vi "RT Loop - Acquire camera_data_1.vi"(8 "Boolean":bool, 11 "Message Queue":refnum<queue>) -> ()   [LabVIEW 2017]
uses:
  UI Error Handlers/support/Message Queue/Message Cluster.ctl
  <vilib>/userdefined/High Color/IMAQdx.ctl
  <vilib>/vision/Avi.llb/IMAQ AVI2 Codec Path.ctl
  <vilib>/vision/Avi.llb/IMAQ AVI2 Refnum.ctl
  Globals/Global - All RT Loop Stop.vi
  Globals/Global - Configuration Options.vi
  <vilib>/vision/driver/NI_Vision_Acquisition_Software.lvlib
  UI Error Handlers/support/Message Queue/Message Queue.lvlib
panel:
  out "Acceleration Log Folder":path=path "/home/lvuser/Log/logfiles_deploy"
  out "Codec Names":string[](array[string])
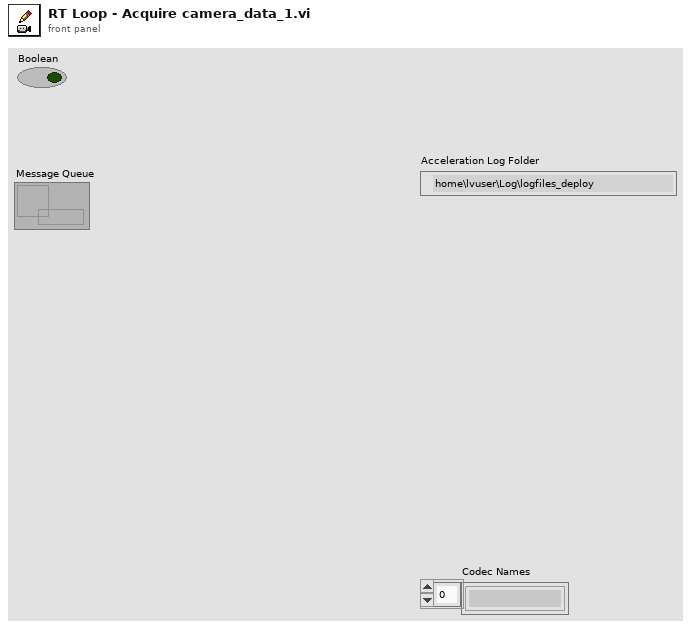
[diagram p1: front panel]
types:
  T1 = typedef "IMAQdx.ctl" = refnum<k21>
  T2 = typedef "Image Type" = u32
  T3 = typedef "IMAQ Image.ctl" = refnum<image>
  T4 = typedef "IMAQ AVI2 Refnum.ctl" = refnum<k20>
  T5 = typedef "IMAQ AVI2 Codec Path.ctl" = u32
  T6 = cluster{"Tool data":cluster{"Number of teeth":sgl}, "Cutting data":cluster{"rpm":sgl}, "Limits":cluster{"Magnitude threshold":sgl, "Tolerance":sgl}, "G1 status":cluster{"G1 trigger":bool}}
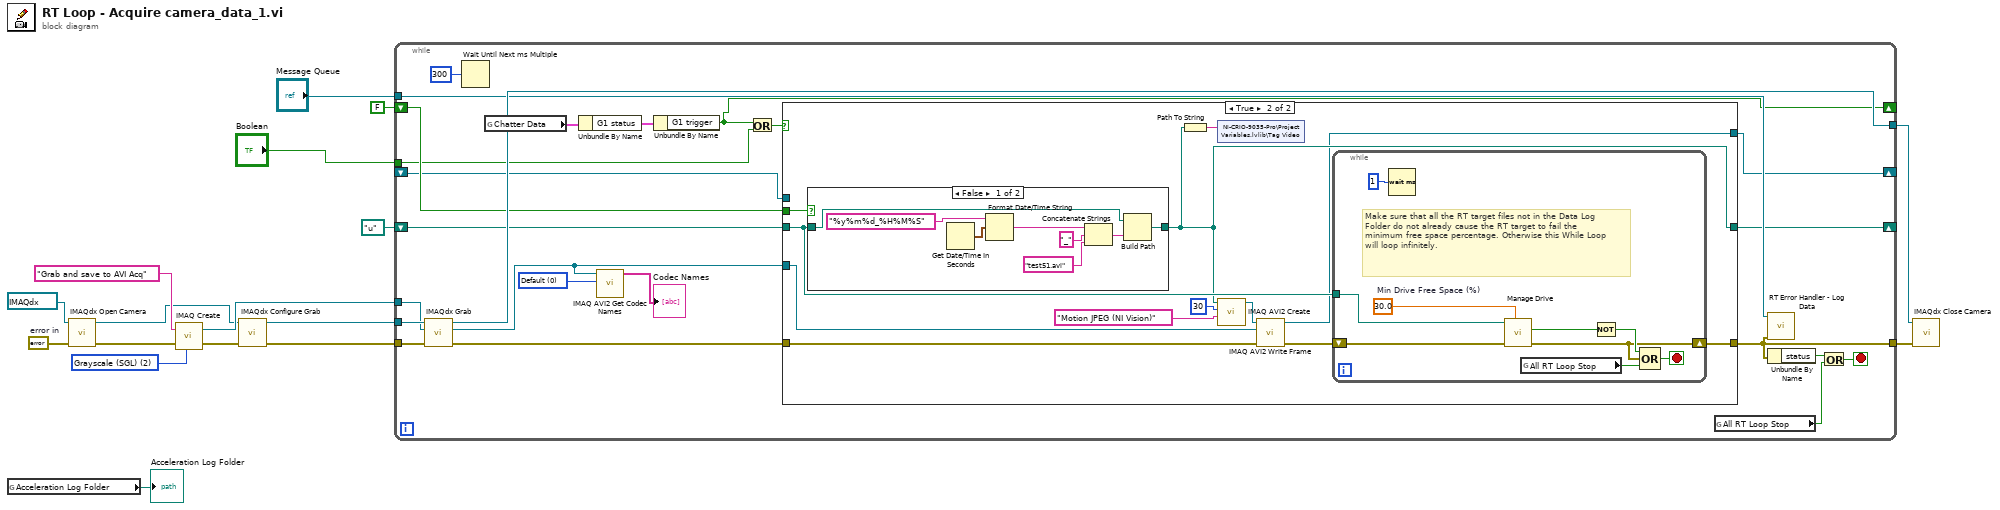
[diagram p0: block diagram]
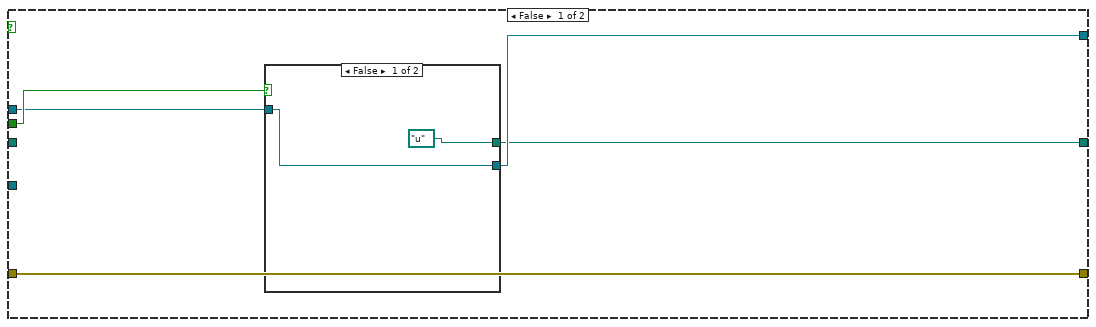
[diagram p2: hidden frame]
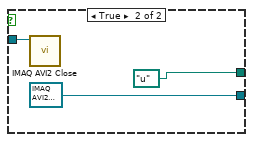
[diagram p3: hidden frame]
diagram:
  w13 = T2 2 items=["Grayscale (U8)", "Grayscale (I16)", "Grayscale (SGL)", "Complex (CSG)", "RGB (U32)", "HSL (U32)", "RGB (U64)", "Grayscale (U16)"] ("Image Type")
  w11 = errorcluster {"status"=FALSE, "code"=0, "source"=""}  # error in
  n1 = global read "Global - Configuration Options.vi" "Acceleration Log Folder"() -> (→"Acceleration Log Folder":path)
  n2 = call <vilib>:"IMAQdx Open Camera.vi"("error in"=w11, "Session In"=T1 "cam0") -> ("error out"=w14:errorcluster, "Session Out"=w9:T1)  [unwired: 8 in]
  n3 = call "IMAQ Create"("Image Name"="Grab and save to AVI Acq", "Image Type"=w13, "error in (no error)"=w14) -> ("New Image"=w17:T3, "error out"=w2:errorcluster)  [unwired: 2 in]
  n4 = call <vilib>:"IMAQdx Configure Grab.vi"("error in"=w2, "Session In"=w9) -> ("error out"=w16:errorcluster, "Session Out"=w15:T1)  [unwired: 8 in]
  n5 = while {
    tunnel: w16 -> [w41]
    tunnel: w15 -> [w40]
    tunnel: w17 -> [w39]
    tunnel: [w27] -> w7
    tunnel: [w38] -> w8
    tunnel: "Message Queue" -> [w28]
    shift-right: [w18] -> _
    shift-left: FALSE ("G1 trigger") -> [w23]
    shift-right: [w22] -> _
    shift-left: path "u:/" ("AVI Path") -> [w30]
    shift-right: [w21] -> _
    shift-left: _ -> [w20]
    tunnel: "Boolean" -> [w19]
    stop <- w35 stop-if-true
    w34 = T5 0 items=["Default", "System", "Built in Vision"] ("Codec Source")
    n6 = call <vilib>:"IMAQdx Grab.vi"("error in"=w41, "Image In"=w39, "Session In"=w40) -> ("error out"=w31:errorcluster, "Image Out"=w32:T3, "Session Out"=w38:T1)  [unwired: 5 in, 1 out]
    n7 = Wait Until Next ms Multiple(millisecond multiple=u32 300 ("milliseconds to wait")) -> ()  [unwired: 1 out]
    n8 = global read "Global - Configuration Options.vi" "Chatter Data"() -> (w26:T6)
    n9 = Unbundle By Name(w26) -> ("G1 status"=w25:cluster{"G1 trigger":bool})
    n10 = call "IMAQ AVI2 Get Codec Names"("Codec Source"=w34, "Image"=w32) -> ("Codec Names"=→"Codec Names":string[])  [unwired: 8 in, 1 out]
    n11 = Unbundle By Name(w25) -> ("G1 trigger"=w18:bool)
    n12 = Or(x=w18, y=w19) -> (x .or. y?=w24:bool)
    n13 = case shown="True" w24 {
      tunnel: w32 -> [_ w60]
      tunnel: w31 -> [w46 w58]
      tunnel: [w46 w63] -> w27
      tunnel: w30 -> [_ w62]
      tunnel: w23 -> [w45 w61]
      tunnel: [w42 w53] -> w22
      tunnel: w20 -> [w44 _]
      tunnel: [w43 w52] -> w21
      frame False {
        n14 = case shown="False" w45 {
          tunnel: w44 -> [w48 w51]
          tunnel: [w48 T4 refnum ("AVI Refnum (duplicate)")] -> w43
          tunnel: [path "u:/" ("AVI Path") path "u:/" ("AVI Path")] -> w42
          frame False {
          }
          frame True {
            n15 = call "IMAQ AVI2 Close"("AVI Refnum"=w51) -> ()  [unwired: 10 in, 1 out]
          }
        }
      }
      frame True {
        n16 = case shown="False" w61 {
          tunnel: w62 -> [w65 w72]
          tunnel: [w64 w72] -> w53
          frame False {
            n17 = Get Date/Time In Seconds() -> (seconds since 1Jan1904=w67:timestamp)
            n18 = Format Date/Time String(time format string (%c)="%y%m%d_%H%M%S", seconds (now)=w67) -> (date/time string=w68:string)  [unwired: 1 out]
            n19 = Concatenate Strings(w68, "_" ("string"), "test51.avi" ("name or relative path")) -> (w71:string)
            n20 = Build Path(base path=w65, name or relative path=w71) -> (appended path=w64:path)
          }
          frame True {
          }
        }
        n21 = Path To String(path=w53) -> (string=w57:string)
        n22 = shared-variable "NI-CRIO-9035-Pro\\Project Variables.lvlib\\Tag Video"(w57) -> ()  [unwired: 1 in, 1 out]
        n23 = call "IMAQ AVI2 Create"("Codec"="Motion JPEG (NI Vision)", "Frames Per Second"=u32 30, "AVI Path"=w53) -> ("AVI Refnum"=w54:T4)  [unwired: 7 in, 1 out]
        n24 = call "IMAQ AVI2 Write Frame"("error in (no error)"=w58, "Image"=w60, "AVI Refnum"=w54) -> ("error out"=w59:errorcluster, "AVI Refnum (duplicate)"=w52:T4)  [unwired: 6 in, 1 out]
        n25 = while {
          shift-right: [w76] -> w63
          shift-left: w59 -> [w77]
          tunnel: w62 -> [w74]
          stop <- w81 stop-if-true
          w75 = 30.0  # Min Drive Free Space (%)
          # "Make sure that all the RT target files not in the Data Log Folder do not already cause the RT target to fail the minimum free space percentage. Otherwise this While Loop will loop infinitely."
          n26 = Wait (ms)(milliseconds to wait=u32 1) -> ()  [unwired: 1 out]
          n27 = call "Manage Drive.vi"("Min Drive Free Space (%)"=w75, "error in"=w77, "Data Folder"=w74) -> ("error out"=w76:errorcluster, "Drive Space Below Limit"=w73:bool)  [unwired: 7 in]
          n28 = global read "Global - All RT Loop Stop.vi" "All RT Loop Stop"() -> (w78:bool)
          n29 = Not(x=w73) -> (.not. x?=w80:bool)
          n30 = Compound Arithmetic op=OR(w80, w76, w78) -> (w81:bool)
        }
      }
    }
    n31 = global read "Global - All RT Loop Stop.vi" "All RT Loop Stop"() -> (w29:bool)
    n32 = call "RT Error Handler - Log Data.vi"("error in (no error)"=w27, "Message Queue"=w28) -> ()  [unwired: 9 in, 1 out]
    n33 = Unbundle By Name(w27) -> ("status"=w36:bool)
    n34 = Or(x=w36, y=w29) -> (x .or. y?=w35:bool)
  }
  n35 = call <vilib>:"IMAQdx Close Camera.vi"("error in"=w7, "Session In"=w8) -> ()  [unwired: 9 in, 1 out]
